vi "createControl.vi"(8 "error in (no error)":errorcluster, 10 "name":string="SALTOPIC", 11 "TypeConstructor in":refnum<class "TypeConstructor.lvclass">) -> (0 "error out":errorcluster, 3 "TypeConstructor out":refnum<class "TypeConstructor.lvclass">)   [LabVIEW 2018, in "TypeConstructor.lvclass"]
uses:
  TypeConstructor.lvclass
  TypeConstructor.lvclass/TypeConstructor.ctl
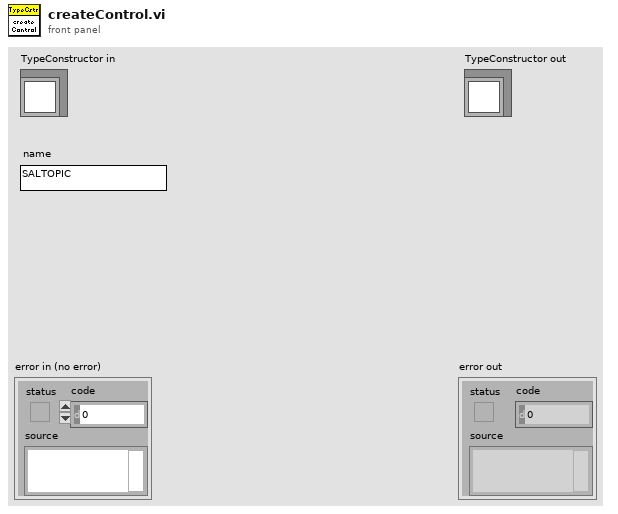
[diagram p1: front panel]
types:
  T1 = enum32{"not a control VI", "control", "typedef", "strict typedef"}
  T2 = enum32{"invalid VI type", "Standard VI", "Control VI", "Global VI", "Polymorphic VI", "Configuration VI", "SubSystem", "Facade VI", "Method VI", "Statechart Diagram VI"}
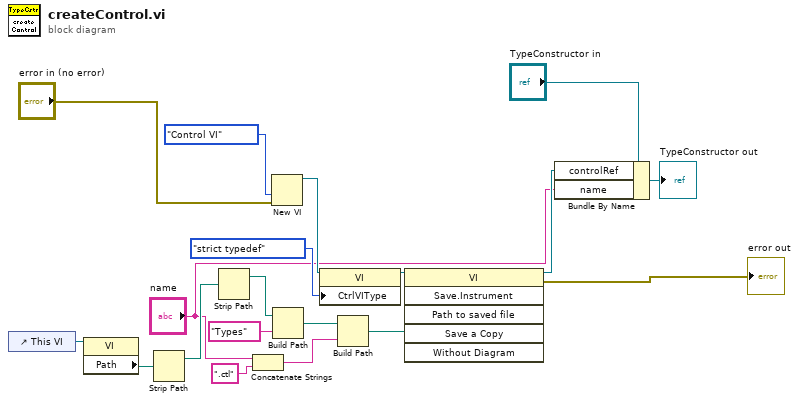
[diagram p0: block diagram]
diagram:
  n1 = control-ref of="This VI"() -> (w16:refnum<vi>)
  n2 = property class="VI"(reference=w16) -> ("Path"=w15:path)  [unwired: 1 in, 2 out]
  n3 = Strip Path(path=w15) -> (stripped path=w14:path)  [unwired: 1 out]
  n4 = Strip Path(path=w14) -> (stripped path=w13:path)  [unwired: 1 out]
  n5 = Concatenate Strings("name", ".ctl" ("string")) -> (w9:string)
  n6 = New VI(8:"error in (no error)", 9:T2."Control VI" ("vi type (standard vi)")) -> (3:w4:refnum<vi>)  [unwired: 5 in, 1 out]
  n7 = Build Path(base path=w13, name or relative path="Types") -> (appended path=w11:path)
  n8 = property class="VI"(reference=w4, "CtrlVIType"=T1."strict typedef" ("Control VI Type")) -> (reference out=w2:refnum<vi>)  [unwired: 1 in, 1 out]
  n9 = Build Path(base path=w11, name or relative path=w9) -> (appended path=w8:path)
  n10 = invoke class="VI" method="Save.Instrument"(reference=w2, "Path to saved file"=w8) -> (reference out=w7:refnum<vi>, error out=→"error out":errorcluster)  [unwired: 4 in, 4 out]
  n11 = Bundle By Name(cluster="TypeConstructor in", "controlRef"=w7, "name"="name") -> (→"TypeConstructor out":refnum<class "TypeConstructor.lvclass">)
